vi "Цифровой пример.vi"() -> ()   [LabVIEW 2017]
doc: "This VI is an exercise in the LabVIEW Basics I course."
panel:
  in  "stop":bool
  in  "Цифровой порт 0":bool[](array[boolean])=[FALSE, FALSE, FALSE, FALSE]
  # "3"
  # "2"
  # "1"
  # "0"
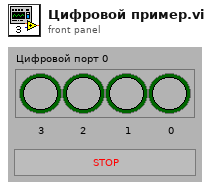
[diagram p1: front panel]
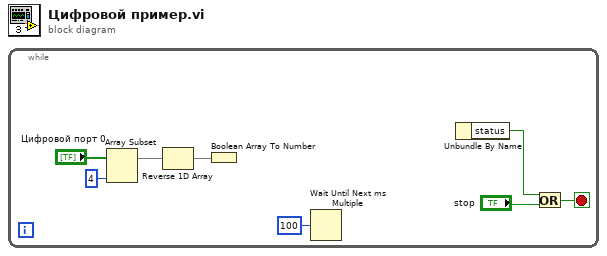
[diagram p0: block diagram]
diagram:
  n1 = while {
    stop <- w3 stop-if-true
    n2 = Array Subset "Array Subset"(array="Цифровой порт 0", length=4) -> (w5:bool[])  [unwired: 1 in]
    n3 = Reverse 1D Array(array=w5) -> (reversed array=w4:bool[])
    n4 = Boolean Array To Number(Boolean array=w4) -> ()  [unwired: 1 out]
    n5 = Wait Until Next ms Multiple(millisecond multiple=u32 100) -> ()  [unwired: 1 out]
    n6 = Unbundle By Name() -> ("status"=w2:bool)  [unwired: 1 in]
    n7 = Or(x=w2, y="stop") -> (x .or. y?=w3:bool)
  }
